vi "staticUpdate.vi"(8 "error in (no error)":errorcluster, 10 "staticChannelUpdate":T1, 11 "BECHWCBasic in":refnum<class "BECHWCBasic.lvclass">) -> (0 "error out":errorcluster, 3 "BECHWCBasic out":refnum<class "BECHWCBasic.lvclass">)   [LabVIEW 2009, in "Hardware.lvlib" / "HWControllers.lvlib" / "BECHWCBasic.lvclass"]
doc: "Update the output state of a channel to a new value"
uses:
  BECHWCBasic.lvclass
  BECHWCBasic.lvclass/BECHWCBasic.ctl
  Channels/Digital/DigitalOutput.lvclass
  Channels/VoltOutput/AnalogOutput.lvclass
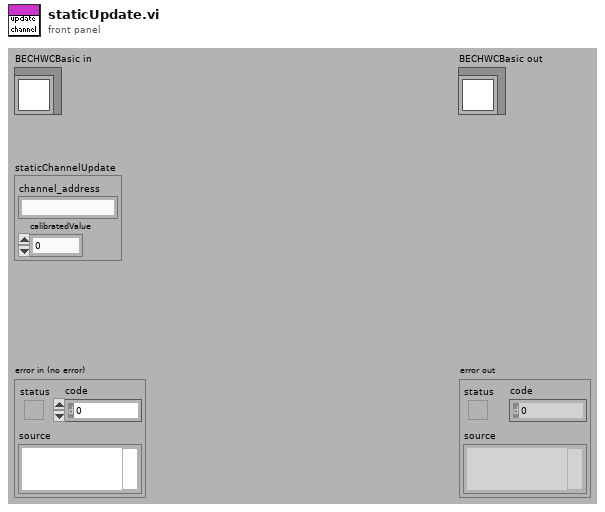
[diagram p1: front panel]
types:
  T1 = cluster{"channel_address":string, "calibratedValue":dbl}
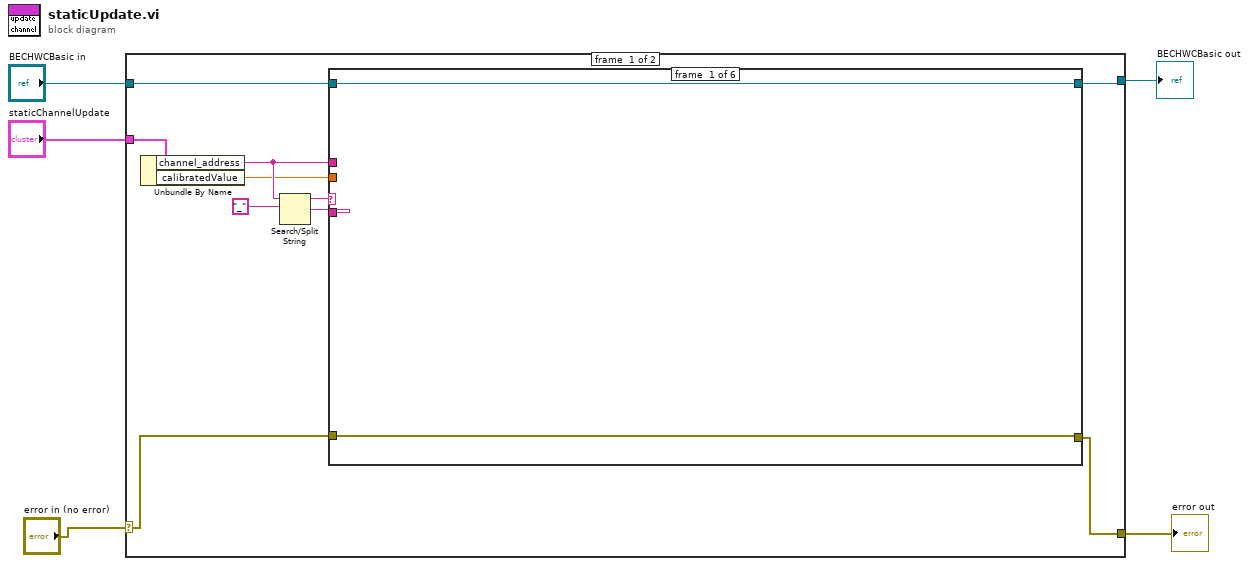
[diagram p0: block diagram]
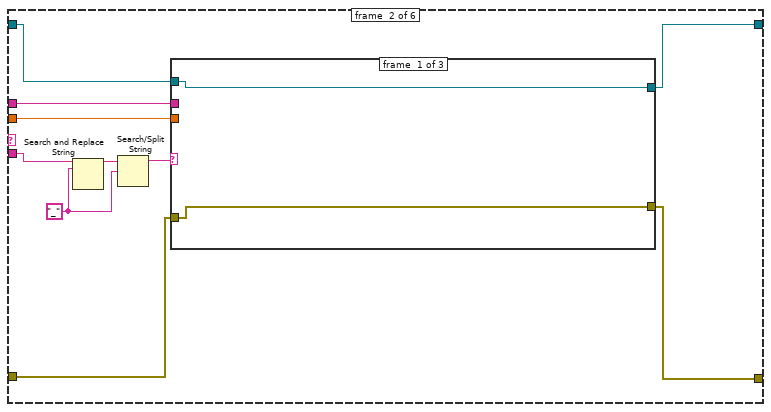
[diagram p2: hidden frame]
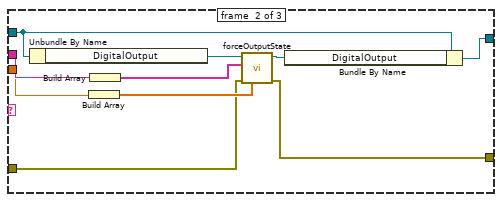
[diagram p3: hidden frame]
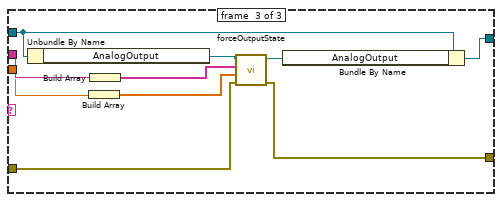
[diagram p4: hidden frame]
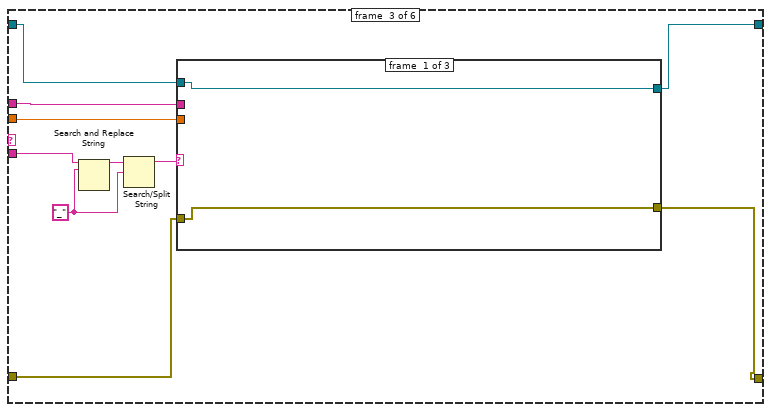
[diagram p5: hidden frame]
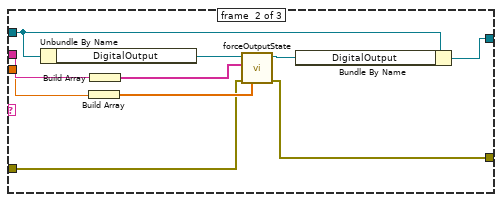
[diagram p6: hidden frame]
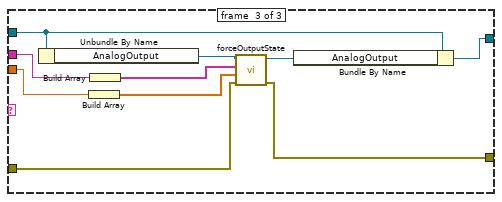
[diagram p7: hidden frame]
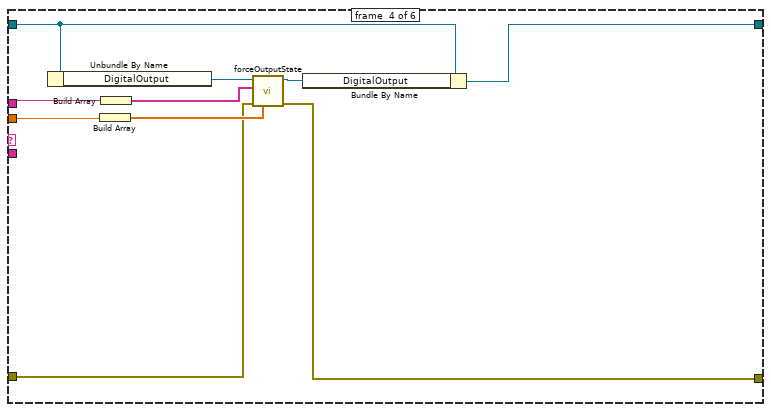
[diagram p8: hidden frame]
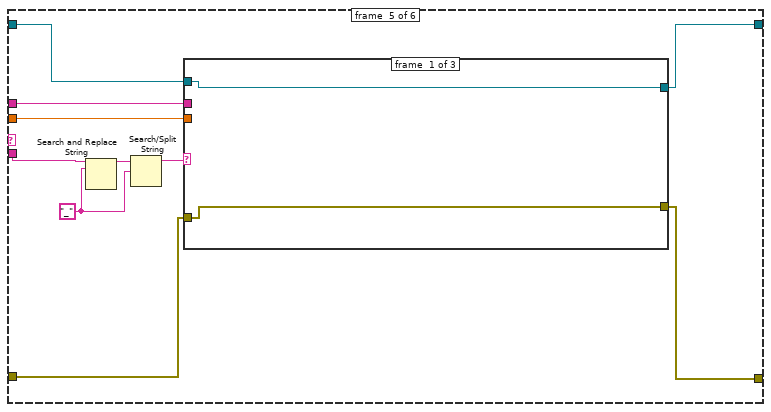
[diagram p9: hidden frame]
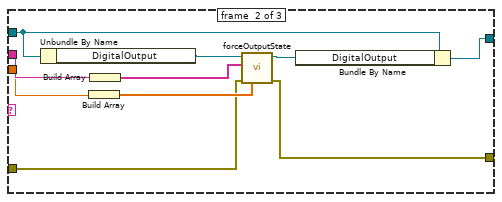
[diagram p10: hidden frame]
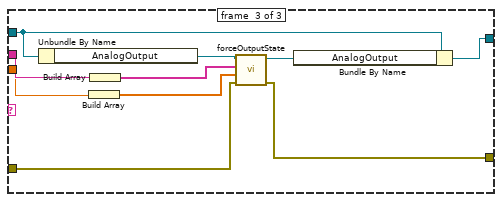
[diagram p11: hidden frame]
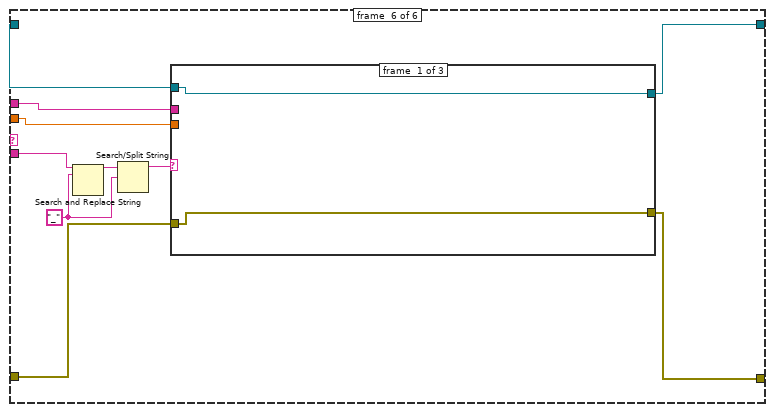
[diagram p12: hidden frame]
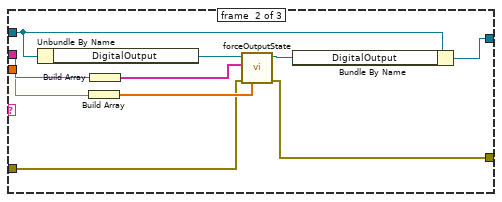
[diagram p13: hidden frame]
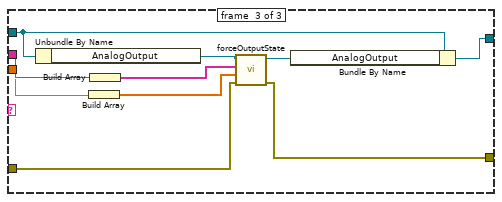
[diagram p14: hidden frame]
diagram:
  n1 = case shown="No Error" "error in (no error)" {
    selector: "error in (no error)" -> [w9 w156]
    tunnel: [w8 w156] -> w4
    tunnel: [w10 w157] -> w1
    tunnel: "BECHWCBasic in" -> [w11 w157]
    tunnel: "staticChannelUpdate" -> [w15 _]
    frame #0 {
      n2 = Unbundle By Name(w15) -> ("channel_address"=w12:string, "calibratedValue"=w7:dbl)
      n3 = Search/Split String(string=w12, search string/char (-)="_") -> (substring before match=w13:string, match + rest of string=w6:string)  [unwired: 1 in, 1 out]
      n4 = case shown="\"Dio64\"" w13 {
        tunnel: w12 -> [_ w24 w56 w90 w100 w127]
        tunnel: w11 -> [w17 w21 w53 w85 w101 w130]
        tunnel: [w17 w20 w52 w83 w94 w129] -> w10
        tunnel: w9 -> [w16 w19 w50 w87 w93 w125]
        tunnel: [w16 w18 w51 w86 w92 w124] -> w8
        tunnel: w7 -> [_ w23 w55 w82 w99 w126]
        tunnel: w6 -> [_ w22 w54 _ w98 w128]
        frame #0 {
        }
        frame #1 {
          w26 = "_"
          n5 = Search and Replace String(input string=w22, search string=w26) -> (result string=w27:string)  [unwired: 6 in, 3 out]
          n6 = Search/Split String(string=w27, search string/char (-)=w26) -> (substring before match=w25:string)  [unwired: 1 in, 2 out]
          n7 = case shown="\"Ao\"" w25 {
            tunnel: w21 -> [w29 w33 w47]
            tunnel: w24 -> [_ w35 w49]
            tunnel: w23 -> [_ w34 w48]
            tunnel: [w29 w32 w46] -> w20
            tunnel: w19 -> [w28 w31 w43]
            tunnel: [w28 w30 w42] -> w18
            frame #0 {
            }
            frame #1 {
              n8 = Unbundle By Name(w33) -> ("DigitalOutput"=w39:refnum<class "DigitalOutput.lvclass">)
              n9 = Build Array(w34) -> (w37:dbl[])
              n10 = Build Array(w35) -> (w38:string[])
              n11 = call-dynamic "forceOutputState.vi"("error in (no error)"=w31, "calibratedValues"=w37, "channel_addresses"=w38, "DigitalOutput in"=w39) -> ("error out"=w30:errorcluster, "DigitalOutput out"=w36:refnum<class "DigitalOutput.lvclass">)  [unwired: 6 in]
              n12 = Bundle By Name(cluster=w33, "DigitalOutput"=w36) -> (w32:refnum<class "BECHWCBasic.lvclass">)
            }
            frame #2 {
              n13 = Unbundle By Name(w47) -> ("AnalogOutput"=w45:refnum<class "AnalogOutput.lvclass">)
              n14 = Build Array(w48) -> (w40:dbl[])
              n15 = Build Array(w49) -> (w41:string[])
              n16 = call-dynamic "forceOutputState.vi"("error in (no error)"=w43, "calibratedValues"=w40, "channel_addresses"=w41, "AnalogOutput in"=w45) -> ("error out"=w42:errorcluster, "AnalogOutput out"=w44:refnum<class "AnalogOutput.lvclass">)  [unwired: 6 in]
              n17 = Bundle By Name(cluster=w47, "AnalogOutput"=w44) -> (w46:refnum<class "BECHWCBasic.lvclass">)
            }
          }
        }
        frame #2 {
          w58 = "_"
          n18 = Search and Replace String(input string=w54, search string=w58) -> (result string=w59:string)  [unwired: 6 in, 3 out]
          n19 = Search/Split String(string=w59, search string/char (-)=w58) -> (substring before match=w57:string)  [unwired: 1 in, 2 out]
          n20 = case shown="\"Ao\"" w57 {
            tunnel: w53 -> [w61 w65 w79]
            tunnel: w56 -> [_ w67 w81]
            tunnel: w55 -> [_ w66 w80]
            tunnel: [w61 w64 w78] -> w52
            tunnel: w50 -> [w60 w63 w75]
            tunnel: [w60 w62 w74] -> w51
            frame #0 {
            }
            frame #1 {
              n21 = Unbundle By Name(w65) -> ("DigitalOutput"=w71:refnum<class "DigitalOutput.lvclass">)
              n22 = Build Array(w66) -> (w69:dbl[])
              n23 = Build Array(w67) -> (w70:string[])
              n24 = call-dynamic "forceOutputState.vi"("error in (no error)"=w63, "calibratedValues"=w69, "channel_addresses"=w70, "DigitalOutput in"=w71) -> ("error out"=w62:errorcluster, "DigitalOutput out"=w68:refnum<class "DigitalOutput.lvclass">)  [unwired: 6 in]
              n25 = Bundle By Name(cluster=w65, "DigitalOutput"=w68) -> (w64:refnum<class "BECHWCBasic.lvclass">)
            }
            frame #2 {
              n26 = Unbundle By Name(w79) -> ("AnalogOutput"=w77:refnum<class "AnalogOutput.lvclass">)
              n27 = Build Array(w80) -> (w72:dbl[])
              n28 = Build Array(w81) -> (w73:string[])
              n29 = call-dynamic "forceOutputState.vi"("error in (no error)"=w75, "calibratedValues"=w72, "channel_addresses"=w73, "AnalogOutput in"=w77) -> ("error out"=w74:errorcluster, "AnalogOutput out"=w76:refnum<class "AnalogOutput.lvclass">)  [unwired: 6 in]
              n30 = Bundle By Name(cluster=w79, "AnalogOutput"=w76) -> (w78:refnum<class "BECHWCBasic.lvclass">)
            }
          }
        }
        frame #3 {
          n31 = Unbundle By Name(w85) -> ("DigitalOutput"=w91:refnum<class "DigitalOutput.lvclass">)
          n32 = Build Array(w82) -> (w88:dbl[])
          n33 = Build Array(w90) -> (w89:string[])
          n34 = call-dynamic "forceOutputState.vi"("error in (no error)"=w87, "calibratedValues"=w88, "channel_addresses"=w89, "DigitalOutput in"=w91) -> ("error out"=w86:errorcluster, "DigitalOutput out"=w84:refnum<class "DigitalOutput.lvclass">)  [unwired: 6 in]
          n35 = Bundle By Name(cluster=w85, "DigitalOutput"=w84) -> (w83:refnum<class "BECHWCBasic.lvclass">)
        }
        frame #4 {
          w96 = "_"
          n36 = Search and Replace String(input string=w98, search string=w96) -> (result string=w97:string)  [unwired: 6 in, 3 out]
          n37 = Search/Split String(string=w97, search string/char (-)=w96) -> (substring before match=w95:string)  [unwired: 1 in, 2 out]
          n38 = case shown="\"Do\"" w95 {
            tunnel: w101 -> [w103 w107 w121]
            tunnel: w100 -> [_ w109 w123]
            tunnel: w99 -> [_ w108 w122]
            tunnel: [w103 w106 w120] -> w94
            tunnel: w93 -> [w102 w105 w117]
            tunnel: [w102 w104 w116] -> w92
            frame #0 {
            }
            frame #1 {
              n39 = Unbundle By Name(w107) -> ("DigitalOutput"=w113:refnum<class "DigitalOutput.lvclass">)
              n40 = Build Array(w108) -> (w111:dbl[])
              n41 = Build Array(w109) -> (w112:string[])
              n42 = call-dynamic "forceOutputState.vi"("error in (no error)"=w105, "calibratedValues"=w111, "channel_addresses"=w112, "DigitalOutput in"=w113) -> ("error out"=w104:errorcluster, "DigitalOutput out"=w110:refnum<class "DigitalOutput.lvclass">)  [unwired: 6 in]
              n43 = Bundle By Name(cluster=w107, "DigitalOutput"=w110) -> (w106:refnum<class "BECHWCBasic.lvclass">)
            }
            frame #2 {
              n44 = Unbundle By Name(w121) -> ("AnalogOutput"=w119:refnum<class "AnalogOutput.lvclass">)
              n45 = Build Array(w122) -> (w114:dbl[])
              n46 = Build Array(w123) -> (w115:string[])
              n47 = call-dynamic "forceOutputState.vi"("error in (no error)"=w117, "calibratedValues"=w114, "channel_addresses"=w115, "AnalogOutput in"=w119) -> ("error out"=w116:errorcluster, "AnalogOutput out"=w118:refnum<class "AnalogOutput.lvclass">)  [unwired: 6 in]
              n48 = Bundle By Name(cluster=w121, "AnalogOutput"=w118) -> (w120:refnum<class "BECHWCBasic.lvclass">)
            }
          }
        }
        frame #5 {
          w132 = "_"
          n49 = Search and Replace String(input string=w128, search string=w132) -> (result string=w133:string)  [unwired: 6 in, 3 out]
          n50 = Search/Split String(string=w133, search string/char (-)=w132) -> (substring before match=w131:string)  [unwired: 1 in, 2 out]
          n51 = case shown="\"Ao\"" w131 {
            tunnel: w130 -> [w135 w139 w153]
            tunnel: w127 -> [_ w141 w155]
            tunnel: w126 -> [_ w140 w154]
            tunnel: [w135 w138 w152] -> w129
            tunnel: w125 -> [w134 w137 w149]
            tunnel: [w134 w136 w148] -> w124
            frame #0 {
            }
            frame #1 {
              n52 = Unbundle By Name(w139) -> ("DigitalOutput"=w145:refnum<class "DigitalOutput.lvclass">)
              n53 = Build Array(w140) -> (w143:dbl[])
              n54 = Build Array(w141) -> (w144:string[])
              n55 = call-dynamic "forceOutputState.vi"("error in (no error)"=w137, "calibratedValues"=w143, "channel_addresses"=w144, "DigitalOutput in"=w145) -> ("error out"=w136:errorcluster, "DigitalOutput out"=w142:refnum<class "DigitalOutput.lvclass">)  [unwired: 6 in]
              n56 = Bundle By Name(cluster=w139, "DigitalOutput"=w142) -> (w138:refnum<class "BECHWCBasic.lvclass">)
            }
            frame #2 {
              n57 = Unbundle By Name(w153) -> ("AnalogOutput"=w151:refnum<class "AnalogOutput.lvclass">)
              n58 = Build Array(w154) -> (w146:dbl[])
              n59 = Build Array(w155) -> (w147:string[])
              n60 = call-dynamic "forceOutputState.vi"("error in (no error)"=w149, "calibratedValues"=w146, "channel_addresses"=w147, "AnalogOutput in"=w151) -> ("error out"=w148:errorcluster, "AnalogOutput out"=w150:refnum<class "AnalogOutput.lvclass">)  [unwired: 6 in]
              n61 = Bundle By Name(cluster=w153, "AnalogOutput"=w150) -> (w152:refnum<class "BECHWCBasic.lvclass">)
            }
          }
        }
      }
    }
    frame #1 {
    }
  }
  "error out" <- w4
  "BECHWCBasic out" <- w1
